vi "Print Error Cleared.vi"(5 "Custom Device? (T)":bool=TRUE, 10 "Your code's public name":string) -> ()   [LabVIEW 2023, in "Ethernet IP Custom Device Custom Device.lvlib"]
doc: "Prints error information out to the console. Provide your code's public name. For example, if your code is about J1939, put that here so the user knows what this printed error information has to do with.\n\nIf this is not a NI VeriStand custom device, write false to the Custom Device? input. This will change the error output.\n\nIf the 'note' field is empty, it is not printed to the console.\n\nExample output 1:\n******J1939 ERROR******\nSource: blah.vi\nCode: 535\n******J1939 ERROR******\n\nExample output 2:\n******XCP and CCP Master CUSTOM DEVICE ERROR******\nSource: blah.vi\nCode: 535\nUser Note: before write\n******XCP and CCP Master CUSTOM DEVICE ERROR******"
uses:
  Ethernet IP Custom Device Custom Device.lvlib
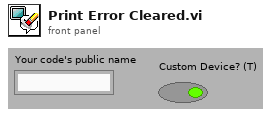
[diagram p1: front panel]
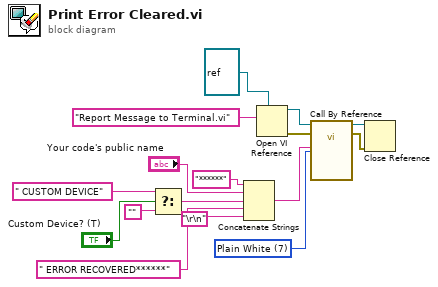
[diagram p0: block diagram]
diagram:
  w5 = u16 7 items=["Plain White"=7, "Bold White"=15, "Bold Blue"=9, "Bold Green"=10, "Bold Red"=12] ("Color (Plain White)")
  n1 = Select(t=" CUSTOM DEVICE" ("String"), s="Custom Device? (T)", f="") -> (s? t:f=w10:string)
  n2 = Concatenate Strings("******" ("String"), "Your code's public name", w10, " ERROR RECOVERED******" ("String"), "\r\n") -> (w4:string)
  n3 = Open VI Reference(type specifier VI Refnum (for type only)=refnum<vi> refnum, vi path="Report Message to Terminal.vi") -> (vi reference=w7:refnum<vi>, error out=w6:errorcluster)  [unwired: 1 in, 3 out]
  n4 = call-by-ref "?"(reference=w7, error in=w6, "Color (Plain White)"=w5, "Message"=w4) -> (reference out=w2:refnum<vi>, error out=w1:errorcluster)  [unwired: 9 in, 1 out]
  n5 = Close Reference(reference=w2, error in (no error)=w1) -> ()  [unwired: 1 out]
